vi "Launch Shape Dialog Core.vi"(6 "Async?":bool, 8 "error in (no error)":errorcluster, 9 "class name":string, 10 "ShapeRef":refnum<data-value>, 11 "Editor Handler in":refnum<class "Image Editor Handler.lvclass">) -> (0 "error out":errorcluster, 3 "Editor Handler out":refnum<class "Image Editor Handler.lvclass">)   [LabVIEW 2017, in "LV Image Editor Framework.lvlib" / "Image Editor Handler.lvclass"]
uses:
  Image Editor Handler.lvclass
  Forms/Shape/Shape.lvclass
  Image Editor Handler.lvclass/Image Editor Handler.ctl
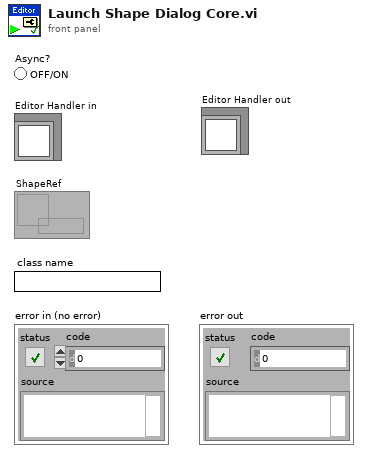
[diagram p1: front panel]
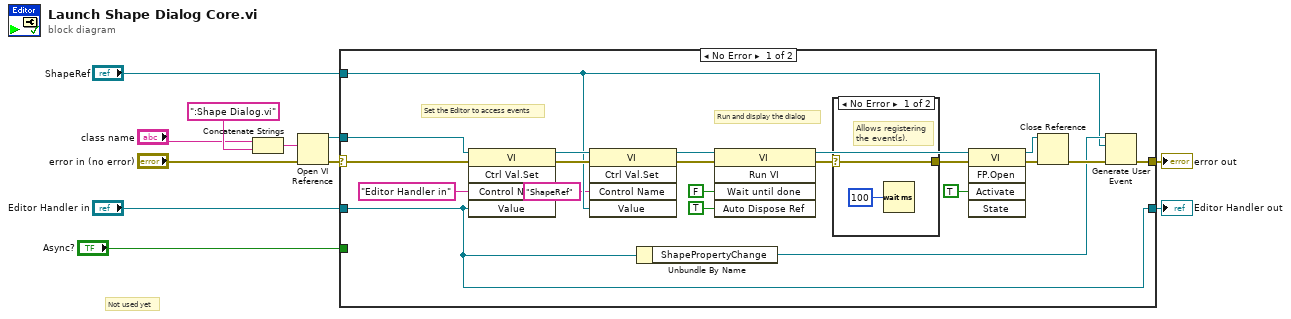
[diagram p0: block diagram]
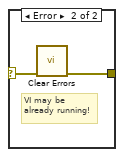
[diagram p2: hidden frame]
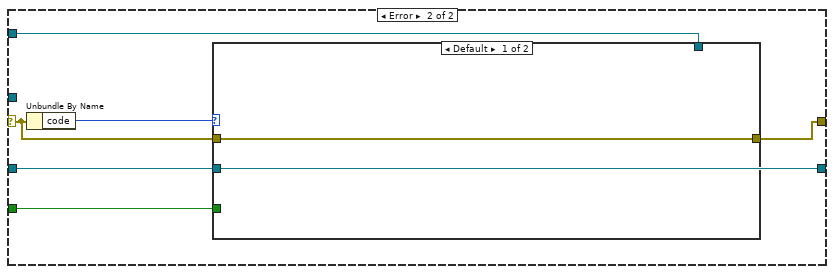
[diagram p3: hidden frame]
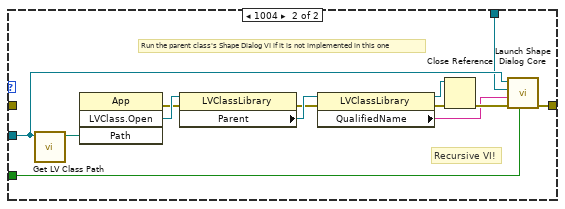
[diagram p4: hidden frame]
diagram:
  # "Not used yet"
  n1 = Concatenate Strings("class name", ":Shape Dialog.vi" ("string")) -> (w3:string)
  n2 = Open VI Reference(vi path=w3, error in (no error)="error in (no error)") -> (vi reference=w6:refnum<vi>, error out=w9:errorcluster)  [unwired: 4 in]
  n3 = case shown="No Error" w9 {
    selector: w9 -> [w27 w37]
    tunnel: "Editor Handler in" -> [w19 w41]
    tunnel: w6 -> [w31 _]
    tunnel: "ShapeRef" -> [w13 w39]
    tunnel: [w29 w38] -> w8
    tunnel: [w19 w41] -> w10
    tunnel: "Async?" -> [_ w40]
    frame No Error {
      # "Run and display the dialog"
      # "Set the Editor to access events"
      n4 = invoke class="VI" method="Ctrl Val.Set"(reference=w31, error in=w27, "Control Name"="Editor Handler in", "Value"=w19) -> (reference out=w17:refnum<vi>, error out=w14:errorcluster)  [unwired: 1 in, 3 out]
      n5 = invoke class="VI" method="Ctrl Val.Set"(reference=w17, error in=w14, "Control Name"="ShapeRef", "Value"=w13) -> (reference out=w16:refnum<vi>, error out=w15:errorcluster)  [unwired: 1 in, 3 out]
      n6 = Unbundle By Name(w19) -> ("ShapePropertyChange"=w18:refnum<user-event>)
      n7 = invoke class="VI" method="Run VI"(reference=w16, error in=w15, "Wait until done"=FALSE ("Wait Until Done"), "Auto Dispose Ref"=TRUE ("Auto Dispose Reference")) -> (reference out=w28:refnum<vi>, error out=w21:errorcluster)  [unwired: 1 in, 3 out]
      n8 = case shown="No Error" w21 {
        selector: w21 -> [w33 w36]
        tunnel: [w33 w35] -> w20
        frame No Error {
          # "Allows registering the event(s)."
          n9 = Wait (ms)(milliseconds to wait=u32 100) -> ()  [unwired: 1 out]
        }
        frame Error {
          # "VI may be already running!"
          n10 = call <vilib>:"Clear Errors.vi"("error in (no error)"=w36) -> ("error out"=w35:errorcluster)  [unwired: 5 in, 1 out]
        }
      }
      n11 = invoke class="VI" method="FP.Open"(reference=w28, error in=w20, "Activate"=TRUE ("Activate?")) -> (reference out=w24:refnum<vi>, error out=w25:errorcluster)  [unwired: 2 in, 3 out]
      n12 = Close Reference(reference=w24, error in (no error)=w25) -> (error out=w30:errorcluster)
      n13 = Generate User Event(user event=w18, event data cluster=w13, error in=w30) -> (error out=w29:errorcluster)  [unwired: 1 in, 1 out]
    }
    frame Error {
      n14 = Unbundle By Name(w37) -> ("code"=w42:i32)
      n15 = case shown="Default" w42 {
        tunnel: w41 -> [_ w47]
        tunnel: w40 -> [_ w45]
        tunnel: w39 -> [_ w46]
        tunnel: [w43 w48] -> w38
        tunnel: w37 -> [w43 _]
        frame Default {
        }
        frame 1004 {
          # "Recursive VI!"
          # "Run the parent class's Shape Dialog VI if it is not implemented in this one"
          n16 = call <vilib>:"Get LV Class Path.vi"("object"=w47) -> ("class path"=w56:path)  [unwired: 9 in, 1 out]
          n17 = invoke class="App" method="LVClass.Open"("Path"=w56) -> (error out=w53:errorcluster, "LVClass.Open"=w55:refnum<vi>)  [unwired: 3 in, 2 out]
          n18 = property class="LVClassLibrary"(reference=w55, error in=w53) -> (error out=w50:errorcluster, "Parent"=w54:refnum<vi>)  [unwired: 1 out]
          n19 = property class="LVClassLibrary"(reference=w54, error in=w50) -> (reference out=w52:refnum<vi>, error out=w51:errorcluster, "QualifiedName"=w44:string)
          n20 = Close Reference(reference=w52, error in (no error)=w51) -> (error out=w49:errorcluster)
          n21 = call "Launch Shape Dialog Core.vi"("Async?"=w45, "error in (no error)"=w49, "class name"=w44, "ShapeRef"=w46, "Editor Handler in"=w47) -> ("error out"=w48:errorcluster)  [unwired: 5 in, 1 out]
        }
      }
    }
  }
  "Editor Handler out" <- w10
  "error out" <- w8
